vi "concat JSON.vi"(8 "error in (no error)":errorcluster, 10 "JSON string 2":string, 11 "JSON string 1":string) -> (0 "error out":errorcluster, 3 "concat JSON string out":string)   [LabVIEW 2018, in "LV-0mq-Julia_roundtrip-lib.lvlib"]
uses:
  LV-0mq-Julia_roundtrip-lib.lvlib
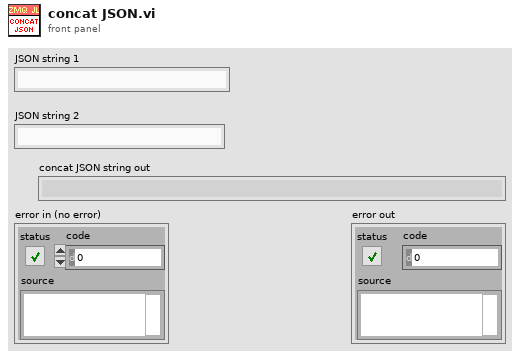
[diagram p1: front panel]
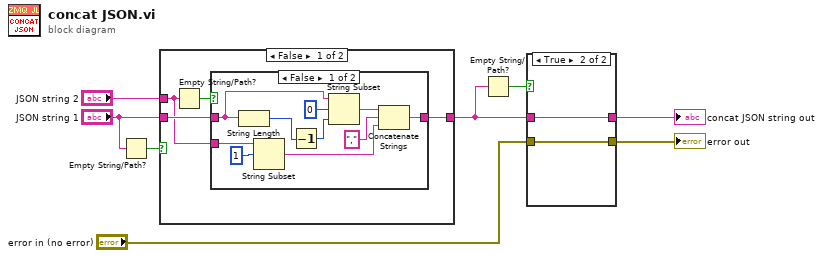
[diagram p0: block diagram]
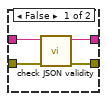
[diagram p2: hidden frame]
diagram:
  n1 = Empty String/Path?(string/path="JSON string 1") -> (empty?=w8:bool)
  n2 = case shown="False" w8 {
    tunnel: [w11 w24] -> w1
    tunnel: "JSON string 2" -> [w9 w24]
    tunnel: "JSON string 1" -> [w10 _]
    frame False {
      n3 = Empty String/Path?(string/path=w9) -> (empty?=w12:bool)
      n4 = case shown="False" w12 {
        tunnel: [w13 w23] -> w11
        tunnel: w10 -> [w22 w23]
        tunnel: w9 -> [w18 _]
        frame False {
          n5 = String Length(string=w22) -> (length=w21:i32)
          n6 = String Subset(string=w18, offset (0)=1) -> (substring=w16:string)  [unwired: 1 in]
          n7 = Decrement(x=w21) -> (x-1=w20:i32)
          n8 = String Subset(string=w22, offset (0)=0, length (rest)=w20) -> (substring=w14:string)
          n9 = Concatenate Strings(w14, "," ("string"), w16) -> (w13:string)
        }
        frame True {
        }
      }
    }
    frame True {
    }
  }
  n10 = Empty String/Path?(string/path=w1) -> (empty?=w2:bool)
  n11 = case shown="True" w2 {
    tunnel: w1 -> [w28 w30]
    tunnel: [w27 w30] -> w5
    tunnel: [w26 w29] -> w4
    tunnel: "error in (no error)" -> [w25 w29]
    frame False {
      n12 = call "check JSON validity.vi"("error in (no error)"=w25, "JSON string in"=w28) -> ("error out"=w26:errorcluster, "JSON string out"=w27:string)  [unwired: 8 in]
    }
    frame True {
    }
  }
  "concat JSON string out" <- w5
  "error out" <- w4
